vi "Request Data JSON.vi"(8 "error in (no error)":errorcluster, 11 "GetProfileParameter in":refnum<class "GetProfileParameter.lvclass">) -> (0 "error out":errorcluster, 2 "Request Data JSON":string, 3 "GetProfileParameter out":refnum<class "GetProfileParameter.lvclass">)   [LabVIEW 2020, in "obs-websocket.lvlib" / "GetProfileParameter.lvclass"]
uses:
  GetProfileParameter.lvclass
  GetProfileParameter.lvclass/GetProfileParameter.ctl
  <vilib>/IlluminatedG/lv-web-crypto/lv-json/JSON/JSON.lvlib
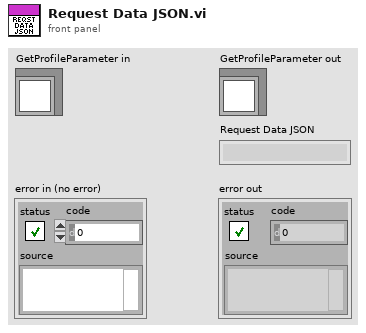
[diagram p1: front panel]
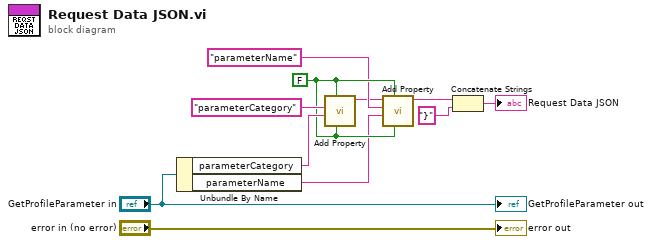
[diagram p0: block diagram]
diagram:
  w7 = FALSE ("Include Empty?")
  n1 = Unbundle By Name("GetProfileParameter in") -> ("parameterCategory"=w8:string, "parameterName"=w5:string)
  n2 = call <vilib>:"Add Property.vi"("String?"=w7, "Include Empty?"=w7, "Value"=w8, "Property Name"="parameterCategory") -> ("String out"=w4:string)  [unwired: 7 in]
  n3 = call <vilib>:"Add Property.vi"("String?"=w7, "Include Empty?"=w7, "Value"=w5, "Property Name"="parameterName", "String In"=w4) -> ("String out"=w3:string)  [unwired: 6 in]
  n4 = Concatenate Strings(w3, "}" ("string")) -> (→"Request Data JSON":string)
  "error out" <- "error in (no error)"
  "GetProfileParameter out" <- "GetProfileParameter in"
